vi "Autoignition McKay-Mark.vi"() -> ()   [LabVIEW 2011]
uses:
  <vilib>/Analysis/NI_AALBase.lvlib
  <vilib>/Analysis/baseanly.llb/Mean (DBL).vi
  <vilib>/Utility/file.llb/Write To Spreadsheet File (DBL).vi
panel:
  out "Data Collection":bool
  in  "file path (dialog if empty)":path=path "c:/temp/trial1"
  in  "?":bool
  out "Waveform Chart":dynamicdata(graph)
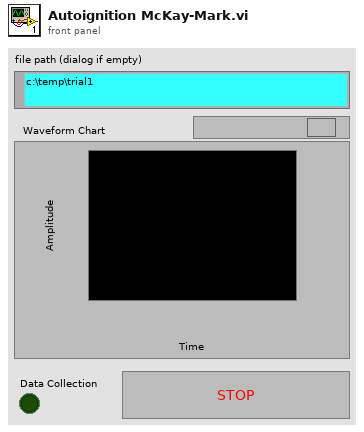
[diagram p1: front panel]
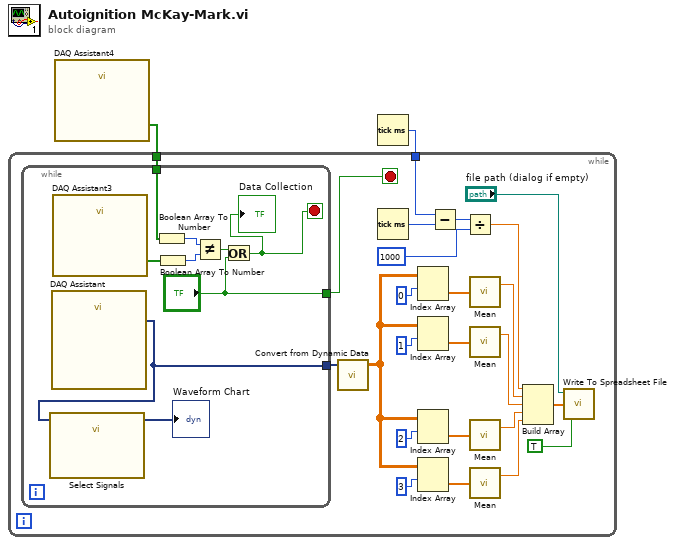
[diagram p0: block diagram]
diagram:
  n1 = call "DAQ Assistant4"() -> ("data"=w2:bool[])  [unwired: 17 in, 2 out]
  n2 = Tick Count (ms)() -> (millisecond timer value=w1:u32)
  n3 = while {
    tunnel: w2 -> [w5]
    tunnel: w1 -> [w3]
    stop <- w17 stop-if-true
    n4 = while {
      tunnel: ["?"] -> w17
      tunnel: w5 -> [w31]
      tunnel: [w30] -> w4
      stop <- w27 stop-if-true
      n5 = call "DAQ Assistant"() -> ("data"=w30:dynamicdata)  [unwired: 17 in, 2 out]
      n6 = call "Select Signals"("Signals"=w30) -> ("Signal Out"=→"Waveform Chart":dynamicdata)  [unwired: 9 in, 1 out]
      n7 = call "DAQ Assistant3"() -> ("data"=w33:bool[])  [unwired: 17 in, 2 out]
      n8 = Boolean Array To Number(Boolean array=w31) -> (number=w34:u32)
      n9 = Boolean Array To Number(Boolean array=w33) -> (number=w35:u32)
      n10 = Not Equal?(x=w34, y=w35) -> (x != y?=w32:bool)
      n11 = Or(x=w32, y="?") -> (x .or. y?=w27:bool)
      "Data Collection" <- w27
    }
    n12 = call "Convert from Dynamic Data"("Dynamic Data Type"=w4) -> ("Array"=w8:dbl[][])  [unwired: 3 in]
    n13 = Tick Count (ms)() -> (millisecond timer value=w7:u32)
    n14 = Index Array(array=w8, index (row)=0) -> (element=w21:dbl[])  [unwired: 1 in]
    n15 = Index Array(array=w8, index (row)=1) -> (element=w22:dbl[])  [unwired: 1 in]
    n16 = Index Array(array=w8, index (row)=2) -> (element=w23:dbl[])  [unwired: 1 in]
    n17 = Index Array(array=w8, index (row)=3) -> (element=w24:dbl[])  [unwired: 1 in]
    n18 = Subtract(x=w3, y=w7) -> (x-y=w6:u32)
    n19 = Divide(x=w6, y=1000) -> (x/y=w18:dbl)
    n20 = call-poly <vilib>:"Mean.vi"("X"=w21) -> ("mean"=w12:dbl)  [unwired: 1 out]
    n21 = call-poly <vilib>:"Mean.vi"("X"=w22) -> ("mean"=w11:dbl)  [unwired: 1 out]
    n22 = call-poly <vilib>:"Mean.vi"("X"=w23) -> ("mean"=w10:dbl)  [unwired: 1 out]
    n23 = call-poly <vilib>:"Mean.vi"("X"=w24) -> ("mean"=w9:dbl)  [unwired: 1 out]
    n24 = Build Array(w18, w12, w11, w10, w9) -> (w25:dbl[])
    n25 = call-poly <vilib>:"Write To Spreadsheet File.vi"("append to file? (new file:F)"=TRUE, "1D data"=w25, "file path (dialog if empty)"="file path (dialog if empty)") -> ()  [unwired: 5 in, 1 out]
  }
